vi "Update String Constants.vi"(8 "error in":errorcluster, 10 "rename data":T3, 11 "vi reference in":refnum<vi>) -> (0 "error out":errorcluster, 2 "rename string constants results":T1[](array[typedef]), 3 "vi reference out":refnum<vi>)   [LabVIEW 2020, in "MeasurementService Editor.lvlib"]
uses:
  MeasurementService Editor.lvlib
  RenameRefactor/Rename Refactor Data.ctl
  RenameRefactor/Rename Refactor Mapping Info.ctl
  RenameRefactor/Rename String Mapping.ctl
  RenameRefactor/Rename String Result.ctl
  RenameRefactor/Rename String.ctl
  <vilib>/Utility/traverseref.llb/TRef TravTarget.ctl
  93bdb3a7-b30e-4ab2-97f7-f3d626629073.vi
  <vilib>/Comparison/Equal/Equal Functor/Equal Functor.lvclass
  <vilib>/Utility/traverseref.llb/VI Scripting - Traverse.lvlib
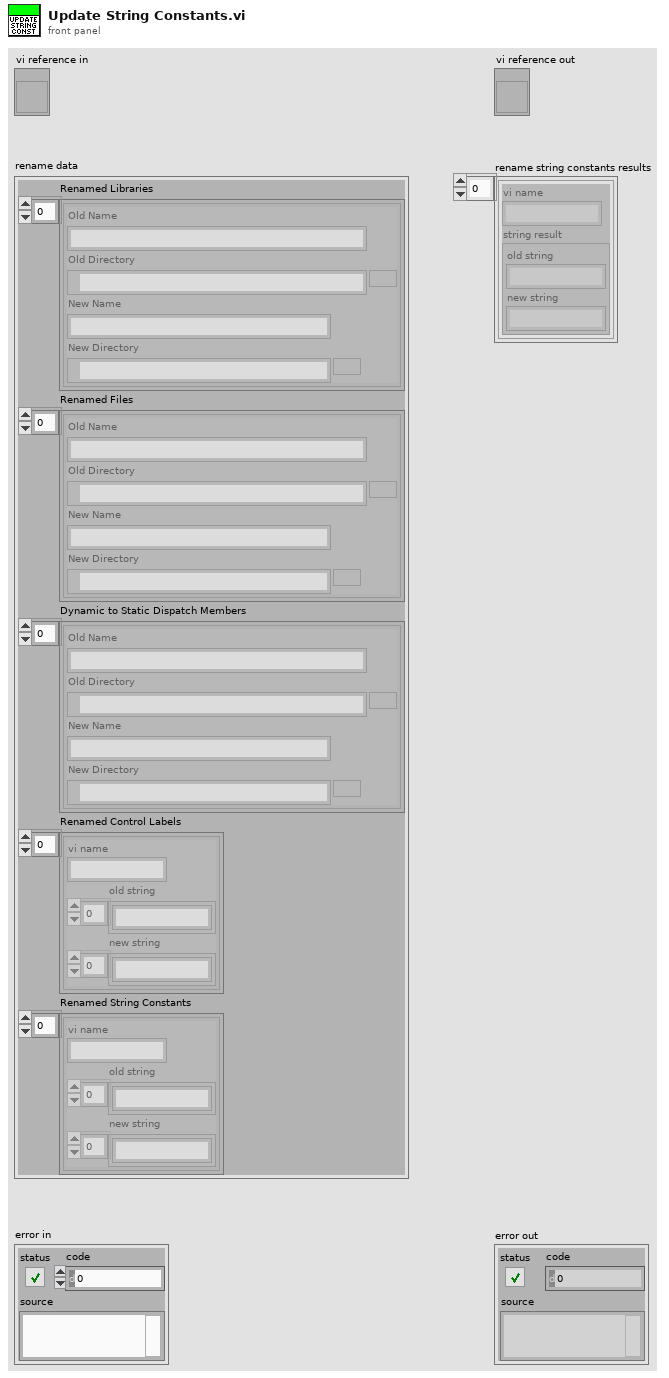
[diagram p1: front panel]
types:
  T1 = typedef "MeasurementService Editor.lvlib/Rename String Result.ctl" = cluster{"vi name":string, "string result":T2}
  T2 = typedef "MeasurementService Editor.lvlib/Rename String.ctl" = cluster{"old string":string, "new string":string}
  T3 = typedef "MeasurementService Editor.lvlib/Rename Refactor Data.ctl" = cluster{"Renamed Libraries":T4[], "Renamed Files":T4[], "Dynamic to Static Dispatch Members":T4[], "Renamed Control Labels":T5[], "Renamed String Constants":T5[]}
  T4 = typedef "MeasurementService Editor.lvlib/Rename Refactor Mapping Info.ctl" = cluster{"Old Name":string, "Old Directory":path, "New Name":string, "New Directory":path}
  T5 = typedef "MeasurementService Editor.lvlib/Rename String Mapping.ctl" = cluster{"vi name":string, "old string":string[], "new string":string[]}
  T6 = typedef "TRef TravTarget.ctl" = enum16{"FP", "BD", "Other"}
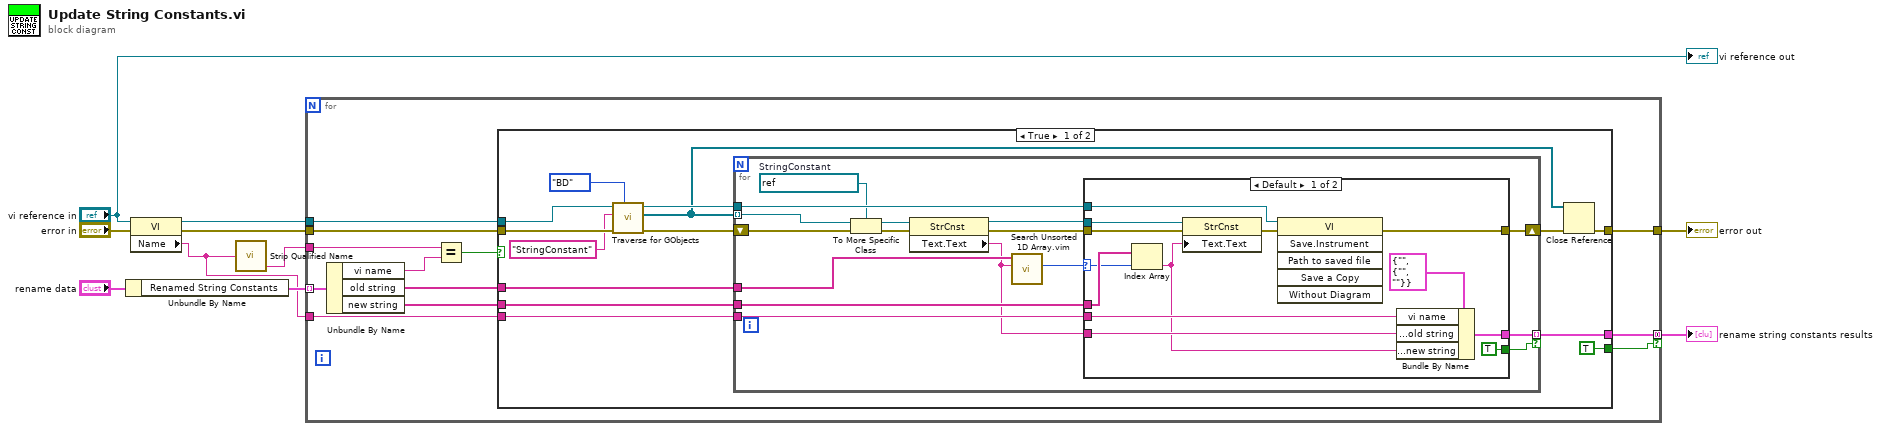
[diagram p0: block diagram]
diagram:
  n1 = Unbundle By Name("rename data") -> ("Renamed String Constants"=w5:T5[])
  n2 = property class="VI"(reference="vi reference in", error in="error in") -> (reference out=w8:refnum<vi>, error out=w7:errorcluster, "Name"=w2:string)
  n3 = call "Strip Qualified Name.vi"("name"=w2) -> ("last name"=w6:string)  [unwired: 5 in, 1 out]
  n4 = for {
    tunnel: w6 -> [w22]
    tunnel: w5 -> [w21] mode=indexing
    tunnel: w8 -> [w19]
    tunnel: w7 -> [w18]
    tunnel: [w14] -> w4
    tunnel: w2 -> [w13]
    tunnel: [w12] -> w1 mode=concatenating if=w11
    n5 = Unbundle By Name(w21) -> ("vi name"=w15:string, "old string"=w17:string[], "new string"=w16:string[])
    n6 = Equal?(x=w22, y=w15) -> (x = y?=w20:bool)
    n7 = case shown="True" w20 {
      tunnel: w19 -> [w36 _]
      tunnel: w18 -> [w35 w67]
      tunnel: [w27 w67] -> w14
      tunnel: w17 -> [w30 _]
      tunnel: w16 -> [w31 _]
      tunnel: w13 -> [w25 _]
      tunnel: [w24 _] -> w12
      tunnel: [TRUE _] -> w11
      frame True {
        n8 = call <vilib>:"Traverse for GObjects.vi"("Traverse Target"=TRef_TravTarget."BD", "error in (no error)"=w35, "Class Name"="StringConstant", "VI Refnum"=w36) -> ("error out"=w32:errorcluster, "References"=w26:refnum<vi>[], "dup VI Refnum"=w29:refnum<vi>)  [unwired: 4 in, 1 out]
        n9 = for {
          tunnel: w26 -> [w52] mode=indexing
          shift-right: [w51] -> w28
          shift-left: w32 -> [w43]
          tunnel: w30 -> [w48]
          tunnel: w31 -> [w46]
          tunnel: w29 -> [w45]
          tunnel: w25 -> [w40]
          tunnel: [w38] -> w24 mode=indexing if=w37
          w41 = refnum<vi> refnum  # StringConstant
          n10 = To More Specific Class(target class=w41, reference=w52, error in=w43) -> (specific class reference=w44:refnum<vi>, error out=w42:errorcluster)
          n11 = property class="StrCnst"(reference=w44, error in=w42) -> (reference out=w50:refnum<vi>, error out=w49:errorcluster, "Text.Text"=w39:string)
          n12 = call "Search Unsorted 1D Array.vim"("element"=w39, "unsorted 1D array"=w48) -> ("index of element"=w47:i32)  [unwired: 9 in]
          n13 = case shown="Default" w47 {
            selector: w47 -> [w62 _]
            tunnel: [w59 w66] -> w51
            tunnel: w50 -> [w65 _]
            tunnel: w49 -> [w64 w66]
            tunnel: w46 -> [w63 _]
            tunnel: w45 -> [w60 _]
            tunnel: w40 -> [w57 _]
            tunnel: w39 -> [w56 _]
            tunnel: [w54 _] -> w38
            tunnel: [TRUE _] -> w37
            frame Default {
              n14 = Index Array(array=w63, index=w62) -> (element=w55:string)
              n15 = property class="StrCnst"(reference=w65, error in=w64, "Text.Text"=w55) -> (error out=w61:errorcluster)  [unwired: 1 out]
              n16 = invoke class="VI" method="Save.Instrument"(reference=w60, error in=w61) -> (error out=w59:errorcluster)  [unwired: 4 in, 5 out]
              n17 = Bundle By Name(cluster=T1 {"vi name"="", "string result"={"old string"="", "new string"=""}} ("rename string result"), "vi name"=w57, "string result.old string"=w56, "string result.new string"=w55) -> (w54:T1)
            }
            frame -1 {
            }
          }
        }
        n18 = Close Reference(reference=w26, error in (no error)=w28) -> (error out=w27:errorcluster)
      }
      frame False {
      }
    }
  }
  "error out" <- w4
  "rename string constants results" <- w1
  "vi reference out" <- "vi reference in"
